vi "GDFsetWaveformArrayRefnum.vi"(8 "error in (no error)":errorcluster, 10 "GDFv1.x in":refnum<class "GDFv1.x.lvclass">, 11 "Waveform Array Refnum in":refnum<data-value>) -> (0 "error out":errorcluster, 3 "GDFv1.x out":refnum<class "GDFv1.x.lvclass">)   [LabVIEW 2016, in "GDF File Reader.lvlib" / "GDFv1.x.lvclass"]
uses:
  GDFv1.x.lvclass
  GDFv1.x.lvclass/GDFv1.x.ctl
panel:
  # "This VI is a part of BCI Design library, http://www.ru-bci.org \nCopyright © 2020, Sotnikov Peter, All rights reserved. License: CC BY-NC 4.0"
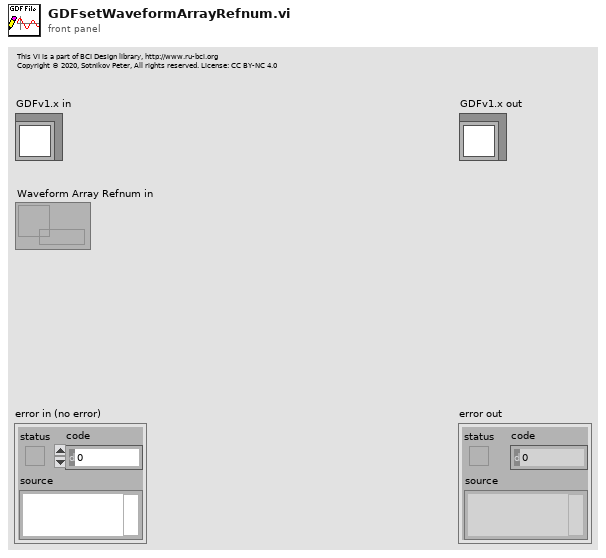
[diagram p1: front panel]
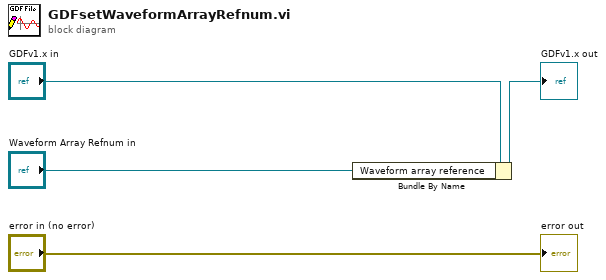
[diagram p0: block diagram]
diagram:
  n1 = Bundle By Name(cluster="GDFv1.x in", "Waveform array reference"="Waveform Array Refnum in") -> (→"GDFv1.x out":refnum<class "GDFv1.x.lvclass">)
  "error out" <- "error in (no error)"
